vi "ShooterOutput.vi"() -> ()   [LabVIEW 2019]
doc: "This VI runs feedback and feedforward control loops, manages safety interlocks, and sends commands to actuators specific to the shooter subsystem."
uses:
  <vilib>/Rock Robotics/WPI/ThirdParty/Phoenix-LabVIEW/Motor Controller/Controls/CTRE_Phoenix_MotorControl_ControlMode.ctl
  <vilib>/Rock Robotics/WPI/Solenoid/WPI_SolenoidValue.ctl
  <vilib>/Rock Robotics/WPI/ThirdParty/Phoenix-LabVIEW/Motor Controller/Controls/CTRE_Phoenix_MotorControl_SupplyCurrentLimitConfiguration.ctl
  b6d1231e-172b-4004-a400-1c444993ac48.vi
  27d7b9d2-eeda-4251-a250-0f206ebe3d42.vi
  refnums.vi
  GRNF_GenericMotor.vi
  GRNF_GenericSolenoid.vi
  sensors.vi
  outputs.vi
  TAI_Solenoid.vi
  TAI_Motor.vi
  dsdata.vi
  <vilib>/Rock Robotics/WPI/Solenoid/WPI_SolenoidSetEnum.vi
  <vilib>/Rock Robotics/WPI/ThirdParty/Phoenix-LabVIEW/Motor Controller/Get/CTRE_Phoenix_MotorController_GetVoltage.vi
panel:
  in  "Plot Kicker":bool
  out "Kicker":T1(graph)
  in  "Kicker PID":T2={"P Gain"=0.0001, "I Gain"=1e-07, "D Gain"=0.01, "F Gain"=0.0002, "I Zone"=200.0, "Min Output"=0.0, "Max Output"=1.0} {"Max Output" min=-1.0 max=1.0 step=0.01; "Min Output" min=-1.0 max=1.0 step=0.01; "I Zone" step=0.01; "F Gain" step=0.01; "D Gain" step=0.01; "I Gain" step=0.01; "P Gain" min=0.0 step=0.01}
  out "Shooter 1":T1(graph)
  in  "Plot Shooter":bool
  out "Shooter 0":T1(graph)
  in  "Shooter PID":T3={"P Gain"=0.0027, "I Gain"=0.0, "D Gain"=0.007, "F Gain"=0.00017, "I Zone"=200.0} {"I Zone" step=0.01; "F Gain" step=0.01; "D Gain" step=0.01; "I Gain" step=0.01; "P Gain" min=0.0 step=0.01}
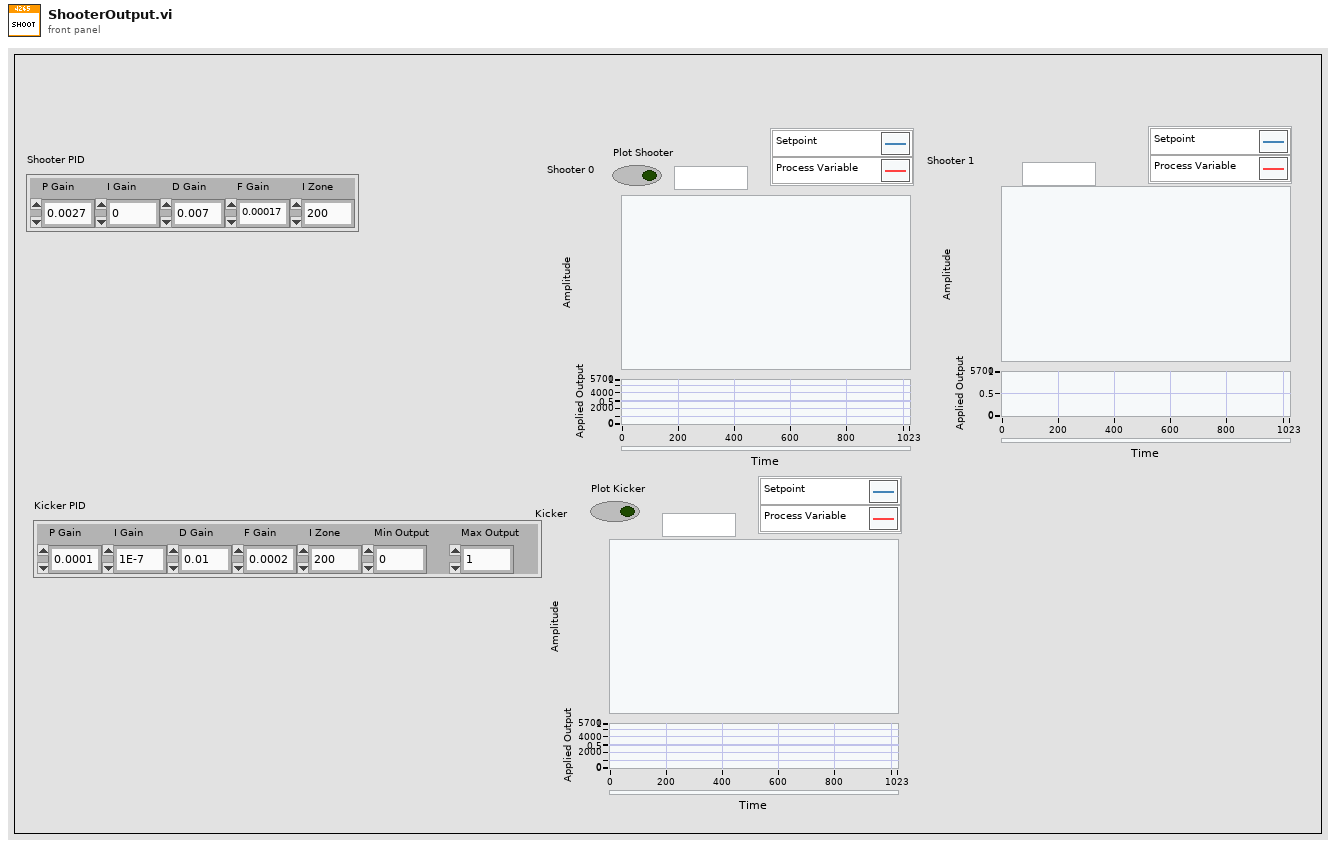
[diagram p1: front panel]
types:
  T1 = cluster{"Sensor Velocity":dbl, "Setpoint":dbl, "Applied Output":dbl}
  T2 = cluster{"P Gain":dbl, "I Gain":dbl, "D Gain":dbl, "F Gain":dbl, "I Zone":dbl, "Min Output":dbl, "Max Output":dbl}
  T3 = cluster{"P Gain":dbl, "I Gain":dbl, "D Gain":dbl, "F Gain":dbl, "I Zone":dbl}
  T4 = typedef "CTRE_Phoenix_MotorControl_ControlMode.ctl" = u16
  T5 = typedef "WPI_MotorControlDeviceRef.ctl" = cluster{"DeviceStatus":errorcluster, "Type":T6, "PWM":cluster{"PWM Channel":T7, "DeadBand":T8}, "CAN":cluster{"Device Number":u8, "SetOutput VI Ref":variant, "GetOutput VI Ref":variant, "Enable VI Ref":variant, "Disable VI Ref":variant, "Data":variant}, "Invert":bool, "DIO PWM":cluster{"PWM \"Enable\" Channel":T7, "DIOChannel":T9, "PWM Rate":dbl}}
  T6 = typedef "WPI_MotorControlType.ctl" = enum16{"PWM", "CAN", "DIO PWM"}
  T7 = typedef "FPGA_DIOPWMChannel.ctl" = enum8{"PWM 0", "PWM 1", "PWM 2", "PWM 3", "PWM 4", "PWM 5", "PWM 6", "PWM 7", "PWM 8", "PWM 9", "PWM MXP 0", "PWM MXP 1", "PWM MXP 2", "PWM MXP 3", "PWM MXP 4", "PWM MXP 5", "PWM MXP 6", "PWM MXP 7", "PWM MXP 8", "PWM MXP 9", "Invalid"}
  T8 = typedef "WPI_PWMDeadband.ctl" = cluster{"Name":string, "maxPositivePwm":i32, "minPositivePwm":i32, "centerPwm":i32, "maxNegativePwm":i32, "minNegativePwm":i32, "angularRange":u16}
  T9 = typedef "FPGA_DIOChannel.ctl" = enum8{"DIO 0", "DIO 1", "DIO 2", "DIO 3", "DIO 4", "DIO 5", "DIO 6", "DIO 7", "DIO 8", "DIO 9", "DIO MXP 0", "DIO MXP 1", "DIO MXP 2", "DIO MXP 3", "DIO MXP 4", "DIO MXP 5", "DIO MXP 6", "DIO MXP 7", "DIO MXP 8", "DIO MXP 9", "DIO MXP 10", "DIO MXP 11", "DIO MXP 12", "DIO MXP 13", "DIO MXP 14", "DIO MXP 15", "SPI Port CS1", "SPI Port CS2", "SPI Port CS3", "SPI Port MISO", "SPI Port MOSI", "Invalid"}
  T10 = typedef "WPI_SolenoidDevRef.ctl" = cluster{"DevStatus":errorcluster, "Pneumatics Control Module":u8, "Forward Solenoid Channel":T11, "Reverse Solenoid Channel":T11}
  T11 = typedef "WPI_SolenoidChannel.ctl" = enum8{"Solenoid 0", "Solenoid 1", "Solenoid 2", "Solenoid 3", "Solenoid 4", "Solenoid 5", "Solenoid 6", "Solenoid 7", "Invalid"}
  T12 = cluster{"P Gain":bool, "I Gain":bool, "D Gain":bool, "F Gain":bool, "I Zone":bool}
  T13 = cluster{"P Gain":bool, "I Gain":bool, "D Gain":bool, "F Gain":bool, "I Zone":bool, "Min Output":bool, "Max Output":bool}
  T14 = typedef "WPI_SolenoidValue.ctl" = enum16{"Off", "On", "Forward", "Reverse"}
  T15 = cluster{"Goal_Kicker_Speed (rpm)":dbl, "Kicker_Speed (rpm)":dbl, "Percent Output":dbl}
  T16 = cluster{"Goal_Shooter_Speed (rpm)":dbl, "Shooter_1_Speed (rpm)":dbl, "Percent Output":dbl}
  T17 = cluster{"Goal_Shooter_Speed (rpm)":dbl, "Shooter_0_Speed (rpm)":dbl, "Percent Output":dbl}
  T18 = typedef "CTRE_Phoenix_MotorControl_SupplyCurrentLimitConfiguration.ctl" = cluster{"Enable?":bool, "Current Limit":dbl, "Threshold Current":dbl, "Threshold Time":dbl}
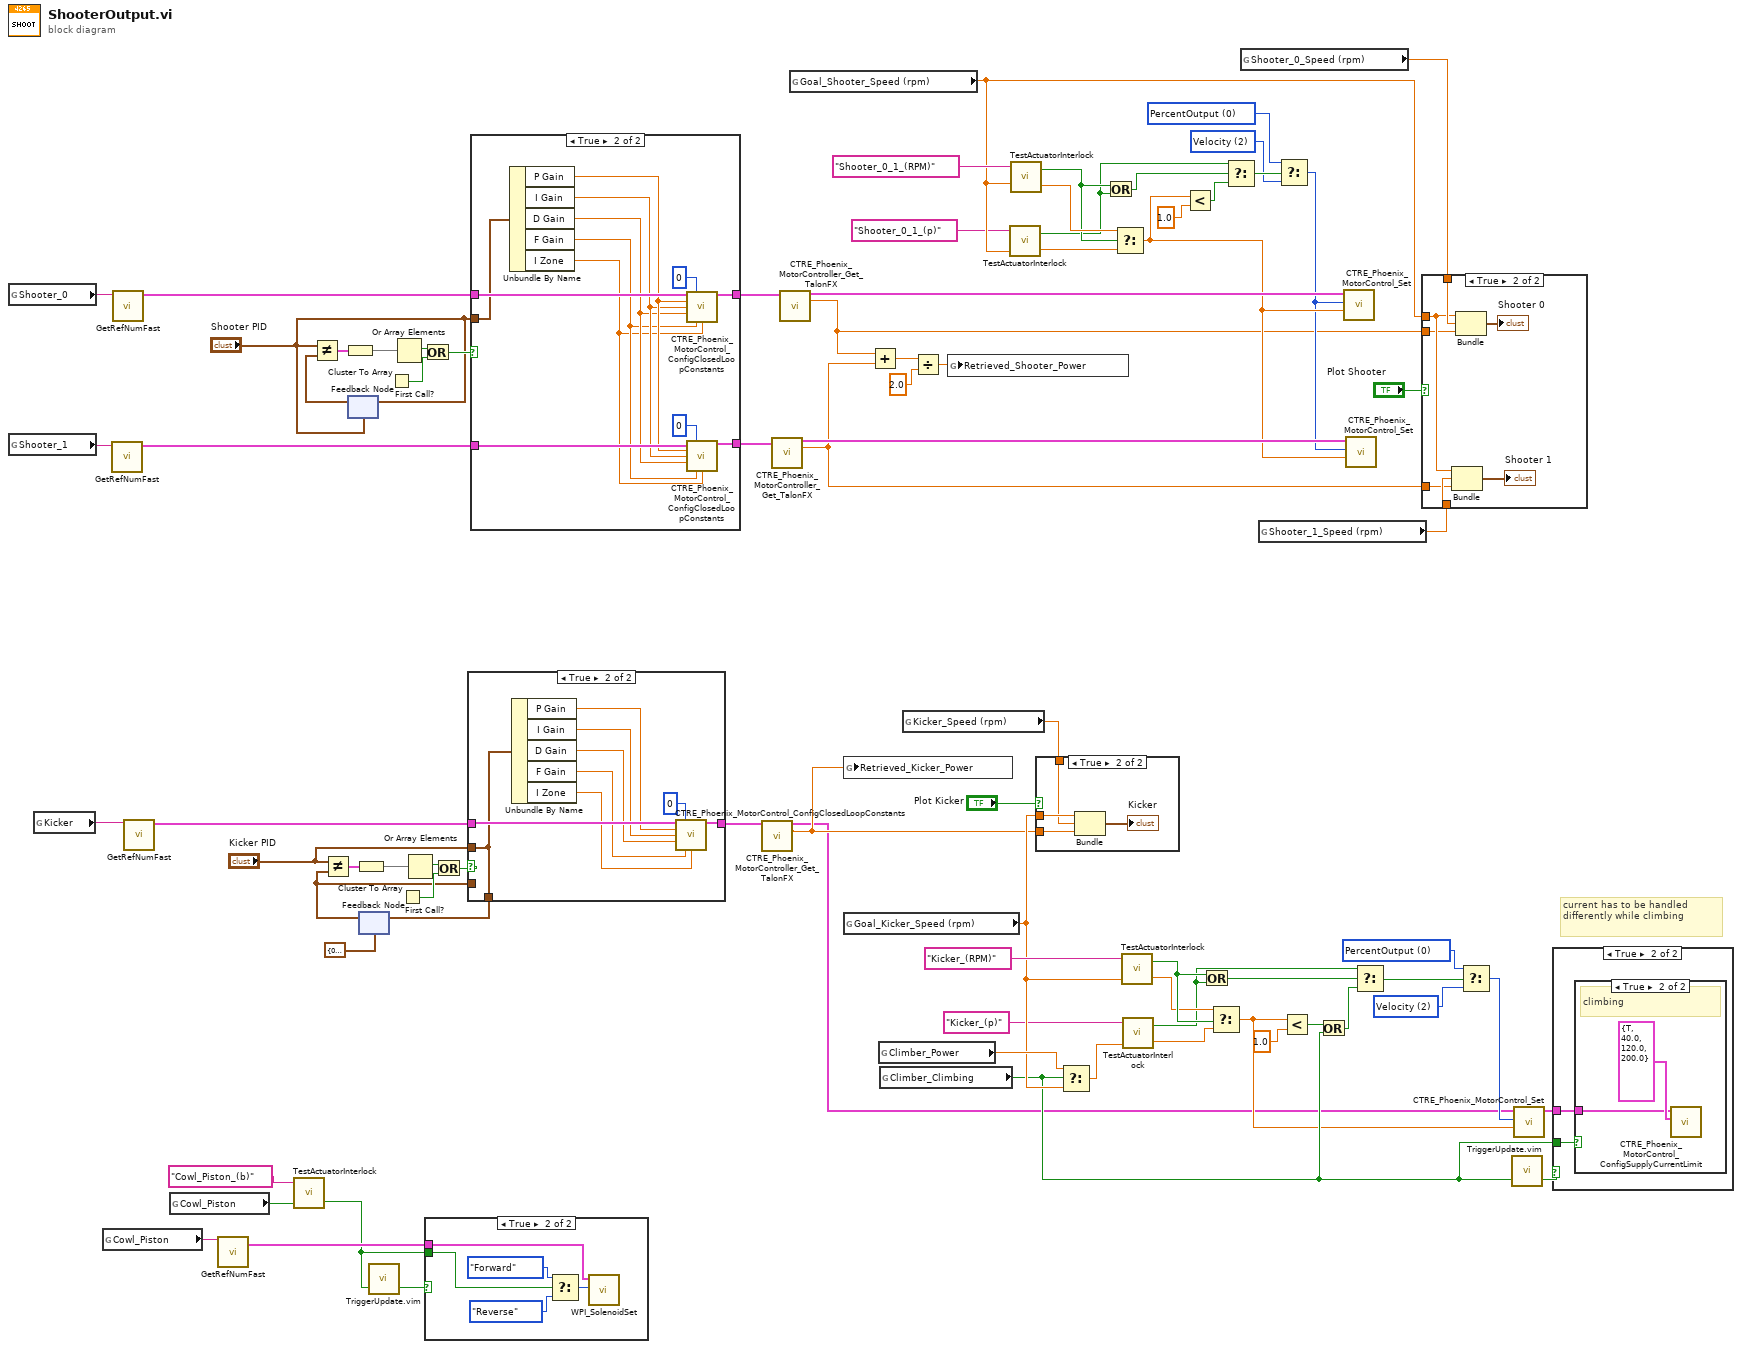
[diagram p0: block diagram]
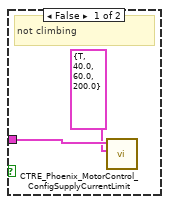
[diagram p4: hidden frame]
diagram:
  w8 = T4 2 items=["PercentOutput"=0, "Position"=1, "Velocity"=2, "Current"=3, "Follower"=5, "MotionProfile"=6, "MotionMagic"=7, "MotionProfileArc"=10, "Disabled"=15] ("Control Mode")
  w9 = T4 0 items=["PercentOutput"=0, "Position"=1, "Velocity"=2, "Current"=3, "Follower"=5, "MotionProfile"=6, "MotionMagic"=7, "MotionProfileArc"=10, "Disabled"=15] ("Control Mode")
  w18 = T4 0 items=["PercentOutput"=0, "Position"=1, "Velocity"=2, "Current"=3, "Follower"=5, "MotionProfile"=6, "MotionMagic"=7, "MotionProfileArc"=10, "Disabled"=15] ("Control Mode")
  w17 = T4 2 items=["PercentOutput"=0, "Position"=1, "Velocity"=2, "Current"=3, "Follower"=5, "MotionProfile"=6, "MotionMagic"=7, "MotionProfileArc"=10, "Disabled"=15] ("Control Mode")
  # "current has to be handled\ndifferently while climbing"
  n1 = global read "refnums.vi" "Shooter_0"() -> (w45:string)
  n2 = global read "refnums.vi" "Shooter_1"() -> (w44:string)
  n3 = global read "refnums.vi" "Kicker"() -> (w43:string)
  n4 = global read "refnums.vi" "Cowl_Piston"() -> (w42:string)
  n5 = call-poly "GetRefNumFast.vi"("RefNum Name"=w44) -> ("Device Reference"=w22:T5)  [unwired: 5 in, 1 out]
  n6 = call-poly "GetRefNumFast.vi"("RefNum Name"=w45) -> ("Device Reference"=w48:T5)  [unwired: 5 in, 1 out]
  n7 = call-poly "GetRefNumFast.vi"("RefNum Name"=w43) -> ("Device Reference"=w47:T5)  [unwired: 5 in, 1 out]
  n8 = global read "outputs.vi" "Cowl_Piston"() -> (w3:bool)
  n9 = call-poly "GetRefNumFast.vi"("RefNum Name"=w42) -> ("Device Reference"=w46:T10)  [unwired: 5 in, 1 out]
  n10 = call-poly "TestActuatorInterlock.vi"("Normal Output"=w3, "Actuator Name"="Cowl_Piston_(b)" ("Actuator_Name")) -> ("Interlock Output"=w4:bool)  [unwired: 1 in, 1 out]
  n11 = feedback #1("Shooter PID") -> (w49:T3)
  n12 = Not Equal?(x="Shooter PID", y=w49) -> (x != y?=w51:T12)
  n13 = Cluster To Array(cluster=w51) -> (array=w50:bool[])
  n14 = feedback-in #1("Shooter PID") -> ()
  n15 = feedback #2(T2 {"P Gain"=0.0, "I Gain"=0.0, "D Gain"=0.0, "F Gain"=0.0, "I Zone"=0.0, "Min Output"=0.0, "Max Output"=0.0} ("PID Constants")) -> (w60:T2)
  n16 = Not Equal?(x="Kicker PID", y=w60) -> (x != y?=w64:T13)
  n17 = Cluster To Array(cluster=w64) -> (array=w63:bool[])
  n18 = call "TriggerUpdate.vim"("Trigger"=w4) -> ("Update"=w59:bool)  [unwired: 2 in]
  n19 = First Call?() -> (First Call?: T/F=w53:bool)
  n20 = Or Array Elements(Boolean array=w50) -> (logical OR=w52:bool)
  n21 = First Call?() -> (First Call?: T/F=w66:bool)
  n22 = Or Array Elements(Boolean array=w63) -> (logical OR=w65:bool)
  n23 = Or(x=w52, y=w53) -> (x .or. y?=w54:bool)
  n24 = case shown="True" w59 {
    tunnel: w4 -> [_ w82]
    tunnel: w46 -> [_ w83]
    frame False {
    }
    frame True {
      n25 = Select(t=WPI_SolenoidValue."Forward" ("Value"), s=w82, f=WPI_SolenoidValue."Reverse" ("Value")) -> (s? t:f=w86:T14)
      n26 = call-poly <vilib>:"WPI_SolenoidSet.vi"("Value"=w86, "SolenoidDevRef"=w83) -> ()  [unwired: 8 in, 2 out]
    }
  }
  n27 = Or(x=w65, y=w66) -> (x .or. y?=w68:bool)
  n28 = case shown="True" w68 {
    tunnel: w47 -> [w87 w96]
    tunnel: "Kicker PID" -> [_ w89]
    tunnel: [w88 w89] -> w61
    tunnel: w60 -> [w88 _]
    tunnel: [w87 w97] -> w13
    frame False {
    }
    frame True {
      n29 = Unbundle By Name(w89) -> ("P Gain"=w95:dbl, "I Gain"=w94:dbl, "D Gain"=w93:dbl, "F Gain"=w92:dbl, "I Zone"=w91:dbl)
      n30 = call <vilib>:"CTRE_Phoenix_MotorControl_ConfigClosedLoopConstants.vi"("PhoenixMotorControlDevRef"=w96, "slotIdx"=0, "P"=w95, "I"=w94, "D"=w93, "F"=w92, "I Zone"=w91) -> ("PhoenixMotorControlDevRef"=w97:T5)  [unwired: 7 in, 1 out]
    }
  }
  n31 = feedback-in #2(w61) -> ()
  n32 = case shown="True" w54 {
    tunnel: w48 -> [w99 w110]
    tunnel: "Shooter PID" -> [_ w109]
    tunnel: [w99 w111] -> w21
    tunnel: [w98 w108] -> w20
    tunnel: w22 -> [w98 w107]
    frame False {
    }
    frame True {
      n33 = Unbundle By Name(w109) -> ("P Gain"=w106:dbl, "I Gain"=w105:dbl, "D Gain"=w104:dbl, "F Gain"=w103:dbl, "I Zone"=w102:dbl)
      n34 = call <vilib>:"CTRE_Phoenix_MotorControl_ConfigClosedLoopConstants.vi"("PhoenixMotorControlDevRef"=w110, "slotIdx"=0, "P"=w106, "I"=w105, "D"=w104, "F"=w103, "I Zone"=w102) -> ("PhoenixMotorControlDevRef"=w111:T5)  [unwired: 7 in, 1 out]
      n35 = call <vilib>:"CTRE_Phoenix_MotorControl_ConfigClosedLoopConstants.vi"("PhoenixMotorControlDevRef"=w107, "slotIdx"=0, "P"=w106, "I"=w105, "D"=w104, "F"=w103, "I Zone"=w102) -> ("PhoenixMotorControlDevRef"=w108:T5)  [unwired: 7 in, 1 out]
    }
  }
  n36 = call-poly <vilib>:"CTRE_Phoenix_MotorController_Get_TalonFX.vi"("PhoenixMotorControlDevRef"=w13) -> ("PhoenixMotorControlDevRef"=w2:T5, "Percent Output"=w12:dbl)  [unwired: 10 in, 3 out]
  n37 = call-poly <vilib>:"CTRE_Phoenix_MotorController_Get_TalonFX.vi"("PhoenixMotorControlDevRef"=w20) -> ("PhoenixMotorControlDevRef"=w16:T5, "Percent Output"=w6:dbl)  [unwired: 10 in, 3 out]
  n38 = call-poly <vilib>:"CTRE_Phoenix_MotorController_Get_TalonFX.vi"("PhoenixMotorControlDevRef"=w21) -> ("PhoenixMotorControlDevRef"=w19:T5, "Percent Output"=w7:dbl)  [unwired: 10 in, 3 out]
  n39 = global read "outputs.vi" "Goal_Shooter_Speed (rpm)"() -> (w38:dbl)
  n40 = global write "sensors.vi" "Retrieved_Kicker_Power"(w12) -> ()
  n41 = global read "outputs.vi" "Goal_Kicker_Speed (rpm)"() -> (w33:dbl)
  n42 = Add(x=w7, y=w6) -> (x+y=w57:dbl)
  n43 = global read "outputs.vi" "Climber_Power"() -> (w78:dbl)
  n44 = global read "outputs.vi" "Climber_Climbing"() -> (w24:bool)
  n45 = global read "sensors.vi" "Kicker_Speed (rpm)"() -> (w70:dbl)
  n46 = Divide(x=w57, y=2.0) -> (x/y=w25:dbl)
  n47 = global write "sensors.vi" "Retrieved_Shooter_Power"(w25) -> ()
  n48 = call-poly "TestActuatorInterlock.vi"("Normal Output"=w38, "Actuator Name"="Shooter_0_1_(p)" ("Actuator_Name")) -> ("Interlock Output"=w35:dbl, "Testing This Actuator"=w36:bool)  [unwired: 1 in]
  n49 = call-poly "TestActuatorInterlock.vi"("Normal Output"=w38, "Actuator Name"="Shooter_0_1_(RPM)" ("Actuator_Name")) -> ("Interlock Output"=w40:dbl, "Testing This Actuator"=w39:bool)  [unwired: 1 in]
  n50 = case shown="True" "Plot Kicker" {
    tunnel: w70 -> [_ w113]
    tunnel: w33 -> [_ w114]
    tunnel: w12 -> [_ w115]
    frame False {
    }
    frame True {
      n51 = Bundle("Goal_Kicker_Speed (rpm)"=w114, "Kicker_Speed (rpm)"=w113, "Percent Output"=w115) -> (→"Kicker":T15)  [unwired: 1 in]
    }
  }
  n52 = Select(t=w78, s=w24, f=w33) -> (s? t:f=w29:dbl)
  n53 = Or(x=w39, y=w36) -> (x .or. y?=w75:bool)
  n54 = Select(t=w40, s=w39, f=w35) -> (s? t:f=w15:dbl)
  n55 = call-poly "TestActuatorInterlock.vi"("Normal Output"=w33, "Actuator Name"="Kicker_(RPM)" ("Actuator_Name")) -> ("Interlock Output"=w31:dbl, "Testing This Actuator"=w32:bool)  [unwired: 1 in]
  n56 = call-poly "TestActuatorInterlock.vi"("Normal Output"=w29, "Actuator Name"="Kicker_(p)" ("Actuator_Name")) -> ("Interlock Output"=w27:dbl, "Testing This Actuator"=w28:bool)  [unwired: 1 in]
  n57 = Less?(x=w15, y=1.0) -> (x < y?=w76:bool)
  n58 = Or(x=w32, y=w28) -> (x .or. y?=w72:bool)
  n59 = Select(t=w31, s=w32, f=w27) -> (s? t:f=w11:dbl)
  n60 = Select(t=w36, s=w75, f=w76) -> (s? t:f=w77:bool)
  n61 = global read "sensors.vi" "Shooter_0_Speed (rpm)"() -> (w55:dbl)
  n62 = global read "sensors.vi" "Shooter_1_Speed (rpm)"() -> (w56:dbl)
  n63 = Select(t=w18, s=w77, f=w17) -> (s? t:f=w14:T4)
  n64 = Less?(x=w11, y=1.0) -> (x < y?=w79:bool)
  n65 = Or(x=w79, y=w24) -> (x .or. y?=w80:bool)
  n66 = call <vilib>:"CTRE_Phoenix_MotorControl_Set.vi"("Output"=w15, "Control Mode"=w14, "PhoenixMotorControlDevRef"=w19) -> ()  [unwired: 7 in, 2 out]
  n67 = call <vilib>:"CTRE_Phoenix_MotorControl_Set.vi"("Output"=w15, "Control Mode"=w14, "PhoenixMotorControlDevRef"=w16) -> ()  [unwired: 7 in, 2 out]
  n68 = Select(t=w28, s=w72, f=w80) -> (s? t:f=w73:bool)
  n69 = case shown="True" "Plot Shooter" {
    tunnel: w56 -> [_ w122]
    tunnel: w55 -> [_ w121]
    tunnel: w38 -> [_ w120]
    tunnel: w7 -> [_ w119]
    tunnel: w6 -> [_ w118]
    frame False {
    }
    frame True {
      n70 = Bundle("Goal_Shooter_Speed (rpm)"=w120, "Shooter_1_Speed (rpm)"=w122, "Percent Output"=w118) -> (→"Shooter 1":T16)  [unwired: 1 in]
      n71 = Bundle("Goal_Shooter_Speed (rpm)"=w120, "Shooter_0_Speed (rpm)"=w121, "Percent Output"=w119) -> (→"Shooter 0":T17)  [unwired: 1 in]
    }
  }
  n72 = Select(t=w9, s=w73, f=w8) -> (s? t:f=w10:T4)
  n73 = call "TriggerUpdate.vim"("Trigger"=w24) -> ("Update"=w81:bool)  [unwired: 2 in]
  n74 = call <vilib>:"CTRE_Phoenix_MotorControl_Set.vi"("Output"=w11, "Control Mode"=w10, "PhoenixMotorControlDevRef"=w2) -> ("PhoenixMotorControlDevRef"=w1:T5)  [unwired: 7 in, 1 out]
  n75 = case shown="True" w81 {
    tunnel: w1 -> [_ w124]
    tunnel: w24 -> [_ w123]
    frame False {
    }
    frame True {
      n76 = case shown="True" w123 {
        tunnel: w124 -> [w126 w127]
        frame False {
          # "not climbing"
          n77 = call <vilib>:"CTRE_Phoenix_MotorControl_ConfigSupplyCurrentLimit.vi"("Supply Current Limit Configuration"=T18 {"Enable?"=TRUE, "Current Limit"=40.0, "Threshold Current"=60.0, "Threshold Time"=200.0}, "PhoenixMotorControlDevRef"=w126) -> ()  [unwired: 8 in, 2 out]
        }
        frame True {
          # "climbing"
          n78 = call <vilib>:"CTRE_Phoenix_MotorControl_ConfigSupplyCurrentLimit.vi"("Supply Current Limit Configuration"=T18 {"Enable?"=TRUE, "Current Limit"=40.0, "Threshold Current"=120.0, "Threshold Time"=200.0}, "PhoenixMotorControlDevRef"=w127) -> ()  [unwired: 8 in, 2 out]
        }
      }
    }
  }
